vi "Select Sample Style.vi"(4 "error IN":errorcluster, 7 "Mfr":string) -> (0 "error Out":errorcluster, 3 "SampleStyles":string[](array[string]))   [LabVIEW 2015]
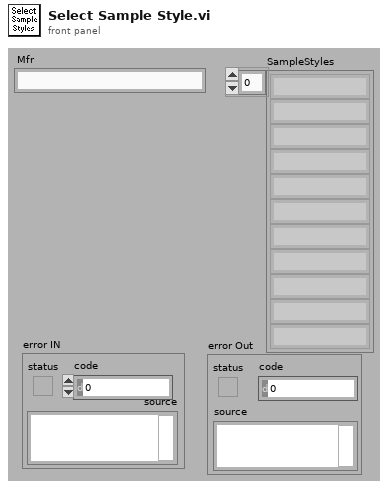
[diagram p1: front panel]
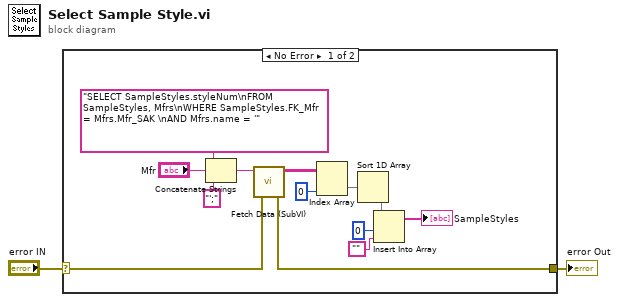
[diagram p0: block diagram]
diagram:
  n1 = case shown="No Error" "error IN" {
    selector: "error IN" -> [w4 w16]
    tunnel: [w3 w16] -> w1
    frame No Error {
      n2 = Concatenate Strings("SELECT SampleStyles.styleNum\nFROM SampleStyles, Mfrs\nWHERE SampleStyles.FK_Mfr = Mfrs.Mfr_SAK \nAND Mfrs.name = '", "Mfr", "';" ("string")) -> (w11:string)
      n3 = call "Fetch Data (SubVI).vi"("error IN"=w4, "query string"=w11) -> ("error OUT"=w3:errorcluster, "recordset data"=w15:string[][])  [unwired: 4 out]
      n4 = Index Array(array=w15, index (col)=0 ("disabled index (col)")) -> (element=w9:string[])  [unwired: 1 in]
      n5 = Sort 1D Array(array=w9) -> (sorted array=w6:string[])
      n6 = Insert Into Array(array=w6, index=0, new element="" ("new element/subarray")) -> (→"SampleStyles":string[])
    }
    frame Error {
    }
  }
  "error Out" <- w1
